vi "SPI to bool.vi"(7 "SCK":u8=15, 8 "error in (no error)":errorcluster, 9 "DO":u8=13, 10 "SPI CS":u8=11, 11 "LINX Resource in":T1) -> (0 "error out":errorcluster, 2 "Array":bool[](array[boolean]), 3 "LINX Resource out":T1)   [LabVIEW 2021]
uses:
  <vilib>/MakerHub/LINX/Private/Type Defs/LINX Ref.ctl
  <vilib>/MakerHub/LINX/Private/Type Defs/Platform.ctl
  <vilib>/MakerHub/LINX/Private/Type Defs/Interface.ctl
  <vilib>/MakerHub/LINX/Private/Device/Type Defs/LINX Device Config.ctl
  <vilib>/MakerHub/LINX/Private/Device/Type Defs/TCP Config.ctl
  <vilib>/MakerHub/LINX/Private/Device/Type Defs/Channels.ctl
  <vilib>/MakerHub/LINX/Public/Peripherals/Digital/Digital Write 1 Chan.vi
  <vilib>/MakerHub/LINX/Public/Peripherals/Digital/Digital Read 1 Chan.vi
  <vilib>/MakerHub/LINX/Public/Peripherals/Digital/Digital Write N Chans.vi
  <vilib>/MakerHub/LINX/Public/Peripherals/Digital/Digital Read N Chans.vi
  <vilib>/MakerHub/LINX/Private/Local IO/LinxDigitalWrite.vi
  <vilib>/MakerHub/LINX/Public/Utilities/Check Channel.vi
  <vilib>/MakerHub/LINX/Private/Local IO/LinxDigitalRead.vi
  <vilib>/MakerHub/LINX/Private/Local IO/Handle Errors.vi
  <vilib>/MakerHub/LINX/Private/Utilties/Generate Error.vi
  <vilib>/MakerHub/LINX/LMH-LINX.lvlib
  <vilib>/MakerHub/LINX/Private/Device/Device.lvlib
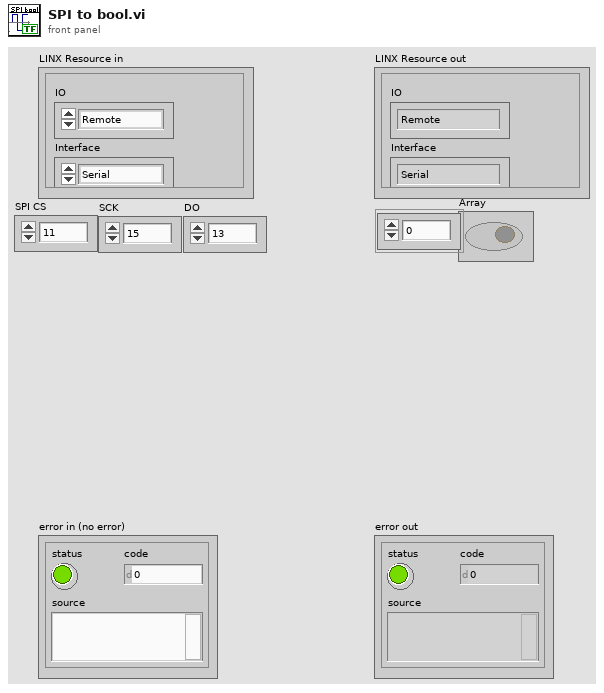
[diagram p1: front panel]
types:
  T1 = typedef "LMH-LINX.lvlib/LINX Ref.ctl" = cluster{"IO":T2, "Interface":T3, "LINX Device Config":T4}
  T2 = typedef "LMH-LINX.lvlib/Platform.ctl" = enum16{"Remote", "Local"}
  T3 = typedef "LMH-LINX.lvlib/Interface.ctl" = enum16{"Serial", "TCP"}
  T4 = typedef "LMH-LINX.lvlib/Device.lvlib/LINX Device Config.ctl" = cluster{"Interface":T3, "COM Port":refnum<visa-resource-name>, "TCP Configuration":T5, "Device Family":u8, "Device ID":u8, "Device Name":string, "TCP Ref":refnum<k5>, "Channels":T6}
  T5 = typedef "LMH-LINX.lvlib/Device.lvlib/TCP Config.ctl" = cluster{"IP Address":string, "Port":u16}
  T6 = typedef "LMH-LINX.lvlib/Channels.ctl" = cluster{"DI":u8[], "DO":u8[], "AI":u8[], "AO":u8[], "PWM":u8[], "QE":u8[], "UART":u8[], "I2C 2":u8[], "SPI":u8[], "CAN":u8[], "Servo":u8[], "AI Ref (V)":dbl, "AI Resolution (Bits)":u8, "AO Ref (V)":dbl, "AO Resolution (Bits)":u8}
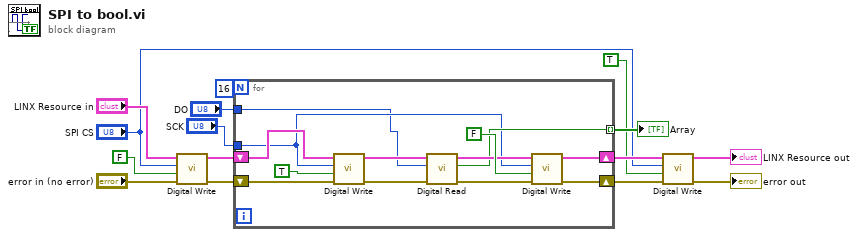
[diagram p0: block diagram]
diagram:
  n1 = call-poly <vilib>:"Digital Write.vi"("Error In"="error in (no error)", "Output Value"=FALSE, "DO Channel"="SPI CS", "LINX Resource"="LINX Resource in") -> ("Error Out"=w8:errorcluster, "LINX Resource"=w7:T1)  [unwired: 6 in]
  n2 = for {
    N: 16 -> [_]
    shift-right: [w20] -> w10
    shift-left: w7 -> [w26]
    shift-right: [w19] -> w11
    shift-left: w8 -> [w25]
    tunnel: [w18] -> w15 mode=indexing
    tunnel: "SCK" -> [w17]
    tunnel: "DO" -> [w16]
    n3 = call-poly <vilib>:"Digital Write.vi"("Error In"=w25, "Output Value"=TRUE, "DO Channel"=w17, "LINX Resource"=w26) -> ("Error Out"=w23:errorcluster, "LINX Resource"=w24:T1)  [unwired: 6 in]
    n4 = call-poly <vilib>:"Digital Read.vi"("Error In"=w23, "DI Channel"=w16, "LINX Resource"=w24) -> ("Error Out"=w21:errorcluster, "DI Value"=w18:bool, "LINX Resource"=w22:T1)  [unwired: 6 in]
    n5 = call-poly <vilib>:"Digital Write.vi"("Error In"=w21, "Output Value"=FALSE, "DO Channel"=w17, "LINX Resource"=w22) -> ("Error Out"=w19:errorcluster, "LINX Resource"=w20:T1)  [unwired: 6 in]
  }
  "Array" <- w15
  n6 = call-poly <vilib>:"Digital Write.vi"("Error In"=w11, "Output Value"=TRUE, "DO Channel"="SPI CS", "LINX Resource"=w10) -> ("Error Out"=→"error out":errorcluster, "LINX Resource"=→"LINX Resource out":T1)  [unwired: 6 in]
